vi "ZVisualize_SingleArrayTesting.vi"() -> ()   [LabVIEW 2016]
uses:
  subVI/ZDataVIS_StateWire.ctl
  <vilib>/Utility/miscctls.llb/LVPointDoubleTypeDef.ctl
panel:
  in  "X Scale Selection":enum32{"Manual", "Auto"}(tab)=enum."Auto"
  in  "Manual CTLs":T1={"X Low"=-0.2, "X High"=-0.1, "X Step Size"=0.001} {"X Step Size" format="%#_6p"; "X High" format="%#_6p"; "X Low" format="%#_6p"}
  in  "Auto CTLs":cluster{"METHOD":bool, "Steps":dbl}={"METHOD"=FALSE, "Steps"=100.0}
  out "XY Graph":cluster{dbl[], dbl[]}[](graph)
  out "Field":dbl=4.108108108108109
  out "slowest":dbl=7.00003046875
  out "2term Intensity":dbl[][](graph)
  in  "X Axis":T2(ring)=enum."dI/dV 2T"
  in  "Y Axis":T2(ring)
  in  "Fake Point Value":dbl format="%#_13g"
  in  "Filter retrieved data? 2":bool=TRUE
  in  "stop":bool
  in  "side points 4T 2":i32=8
  out "side points 4Ttemp":i32=8
  in  "side points 2T 2":i32=12
  out "side points 2Ttemp":i32=12
  in  "side points 4T":i32=8
  in  "side points 2T":i32=12
  in  "Fit Points 2":dbl=10.0
  in  "T/B     third axis":bool
  in  "color scale":u32[](array[colorbox])=[16711680, 16772608, 6618880, 3381759, 16860, 10420479]
  in  "Voffset -2T":dbl=2e-05 format="%#_6p"
  in  "Voffset-4T":dbl=-5e-05 format="%#_4p"
  in  "Field/Temperature":i32(slide) min=0 max=36 step=1
  out "Scan names":string[](array[string])=["DAQ_Vbg", "B", "B"]
  out "Cursor Graph":cluster{dbl[], dbl[]}(graph)={[0.0, 0.0, 0.0, 0.0, 0.0, 0.0, 0.0, 0.0, 0.25, 0.25, 0.25, 0.25, 0.25, 0.25, 0.25, 0.25, 0.5, 0.5, 0.5, 0.5, 0.5, 0.5, 0.5, 0.5, 0.75, 0.75, 0.75, 0.75, 0.75, 0.75, 0.75, 0.75, 1.0, 1.0, 1.0, 1.0, 1.0, 1.0, 1.0, 1.0, 1.25, 1.25, 1.25, 1.25, 1.25, 1.25, 1.25, 1.25, 1.5, 1.5, 1.5, 1.5, 1.5, 1.5, 1.5, 1.5, 1.75, 1.75, 1.75, 1.75, 1.75, 1.75, 1.75, 1.75, 2.0, 2.0, 2.0, 2.0, 2.0, 2.0, 2.0, 2.0, 2.25, 2.25, 2.25, 2.25, 2.25, 2.25, 2.25, 2.25, 2.5, 2.5, 2.5, 2.5, 2.5, 2.5, 2.5, 2.5, 2.75, 2.75, 2.75, 2.75, 2.75, 2.75, 2.75, 2.75, 3.0, 3.0, 3.0, 3.0, 3.0, 3.0, 3.0, 3.0, 3.25, 3.25, 3.25, 3.25, 3.25, 3.25, 3.25, 3.25, 3.5, 3.5, 3.5, 3.5, 3.5, 3.5, 3.5, 3.5, 3.75, 3.75, 3.75, 3.75, 3.75, 3.75, 3.75, 3.75, 4.0, 4.0, 4.0, 4.0, 4.0, 4.0, 4.0, 4.0, 4.25, 4.25, 4.25, 4.25, 4.25, 4.25, 4.25, 4.25, 4.5, 4.5, 4.5, 4.5, 4.5, 4.5, 4.5, 4.5, 4.75, 4.75, 4.75, 4.75, 4.75, 4.75, 4.75, 4.75, 5.0, 5.0, 5.0, 5.0, 5.0, 5.0, 5.0, 5.0, 5.25, 5.25, 5.25, 5.25, 5.25, 5.25, 5.25, 5.25, 5.5, 5.5, 5.5, 5.5, 5.5, 5.5, 5.5, 5.5, 5.75, 5.75, 5.75, 5.75, 5.75, 5.75, 5.75, 5.75, 6.0, 6.0, 6.0, 6.0, 6.0, 6.0, 6.0, 6.0, 6.25, 6.25, 6.25, 6.25, 6.25, 6.25, 6.25, 6.25, 6.5, 6.5, 6.5, 6.5, 6.5, 6.5, 6.5, 6.5, 6.75, 6.75, 6.75, 6.75, 6.75, 6.75, 6.75, 6.75, 7.0, 7.0, 7.0, 7.0, 7.0, 7.0, 7.0, 7.0, 7.25, 7.25, 7.25, 7.25, 7.25, 7.25, 7.25, 7.25, 7.5, 7.5, 7.5, 7.5, 7.5, 7.5, 7.5, 7.5, 7.75, 7.75, 7.75, 7.75, 7.75, 7.75, 7.75, 7.75, 8.0, 8.0, 8.0, 8.0, 8.0, 8.0, 8.0, 8.0, 8.25, 8.25, 8.25, 8.25, 8.25, 8.25, 8.25, 8.25, 8.5, 8.5, 8.5, 8.5, 8.5, 8.5, 8.5, 8.5, 8.75, 8.75, 8.75, 8.75, 8.75, 8.75, 8.75, 8.75, 9.0, 9.0, 9.0, 9.0, 9.0, 9.0, 9.0, 9.0, 9.25, 9.25, 9.25, 9.25, 9.25, 9.25, 9.25, 9.25, 9.5, 9.5, 9.5, 9.5, 9.5, 9.5, 9.5, 9.5, 9.75, 9.75, 9.75, 9.75, 9.75, 9.75, 9.75, 9.75, 10.0, 10.0, 10.0, 10.0, 10.0, 10.0, 10.0, 10.0, 10.25, 10.25, 10.25, 10.25, 10.25, 10.25, 10.25, 10.25, 10.5, 10.5, 10.5, 10.5, 10.5, 10.5, 10.5, 10.5, 10.75, 10.75, 10.75, 10.75, 10.75, 10.75, 10.75, 10.75, 11.0, 11.0, 11.0, 11.0, 11.0, 11.0, 11.0, 11.0, 11.25, 11.25, 11.25, 11.25, 11.25, 11.25, 11.25, 11.25, 11.5, 11.5, 11.5, 11.5, 11.5, 11.5, 11.5, 11.5, 11.75, 11.75, 11.75, 11.75, 11.75, 11.75, 11.75, 11.75, 12.0, 12.0, 12.0, 12.0, 12.0, 12.0, 12.0, 12.0, 12.25, 12.25, 12.25, 12.25, 12.25, 12.25, 12.25, 12.25, 12.5, 12.5, 12.5, 12.5, 12.5, 12.5, 12.5, 12.5, 12.75, 12.75, 12.75, 12.75, 12.75, 12.75, 12.75, 12.75, 13.0, 13.0, 13.0, 13.0, 13.0, 13.0, 13.0, 13.0, 13.25, 13.25, 13.25, 13.25, 13.25, 13.25, 13.25, 13.25, 13.5, 13.5, 13.5, 13.5, 13.5, 13.5, 13.5, 13.5, 13.75, 13.75, 13.75, 13.75, 13.75, 13.75, 13.75, 13.75, 14.0, 14.0, 14.0, 14.0, 14.0, 14.0, 14.0, 14.0, 14.25, 14.25, 14.25, 14.25, 14.25, 14.25, 14.25, 14.25, 14.5, 14.5, 14.5, 14.5, 14.5, 14.5, 14.5, 14.5, 14.75, 14.75, 14.75, 14.75, 14.75, 14.75, 14.75, 14.75, 15.0, 15.0, 15.0, 15.0, 15.0, 15.0, 15.0, 15.0], [0.0, 1.0, 2.0, 3.0, 4.0, 5.0, 6.0, 7.0, 0.0, 1.0, 2.0, 3.0, 4.0, 5.0, 6.0, 7.0, 0.0, 1.0, 2.0, 3.0, 4.0, 5.0, 6.0, 7.0, 0.0, 1.0, 2.0, 3.0, 4.0, 5.0, 6.0, 7.0, 0.0, 1.0, 2.0, 3.0, 4.0, 5.0, 6.0, 7.0, 0.0, 1.0, 2.0, 3.0, 4.0, 5.0, 6.0, 7.0, 0.0, 1.0, 2.0, 3.0, 4.0, 5.0, 6.0, 7.0, 0.0, 1.0, 2.0, 3.0, 4.0, 5.0, 6.0, 7.0, 0.0, 1.0, 2.0, 3.0, 4.0, 5.0, 6.0, 7.0, 0.0, 1.0, 2.0, 3.0, 4.0, 5.0, 6.0, 7.0, 0.0, 1.0, 2.0, 3.0, 4.0, 5.0, 6.0, 7.0, 0.0, 1.0, 2.0, 3.0, 4.0, 5.0, 6.0, 7.0, 0.0, 1.0, 2.0, 3.0, 4.0, 5.0, 6.0, 7.0, 0.0, 1.0, 2.0, 3.0, 4.0, 5.0, 6.0, 7.0, 0.0, 1.0, 2.0, 3.0, 4.0, 5.0, 6.0, 7.0, 0.0, 1.0, 2.0, 3.0, 4.0, 5.0, 6.0, 7.0, 0.0, 1.0, 2.0, 3.0, 4.0, 5.0, 6.0, 7.0, 0.0, 1.0, 2.0, 3.0, 4.0, 5.0, 6.0, 7.0, 0.0, 1.0, 2.0, 3.0, 4.0, 5.0, 6.0, 7.0, 0.0, 1.0, 2.0, 3.0, 4.0, 5.0, 6.0, 7.0, 0.0, 1.0, 2.0, 3.0, 4.0, 5.0, 6.0, 7.0, 0.0, 1.0, 2.0, 3.0, 4.0, 5.0, 6.0, 7.0, 0.0, 1.0, 2.0, 3.0, 4.0, 5.0, 6.0, 7.0, 0.0, 1.0, 2.0, 3.0, 4.0, 5.0, 6.0, 7.0, 0.0, 1.0, 2.0, 3.0, 4.0, 5.0, 6.0, 7.0, 0.0, 1.0, 2.0, 3.0, 4.0, 5.0, 6.0, 7.0, 0.0, 1.0, 2.0, 3.0, 4.0, 5.0, 6.0, 7.0, 0.0, 1.0, 2.0, 3.0, 4.0, 5.0, 6.0, 7.0, 0.0, 1.0, 2.0, 3.0, 4.0, 5.0, 6.0, 7.0, 0.0, 1.0, 2.0, 3.0, 4.0, 5.0, 6.0, 7.0, 0.0, 1.0, 2.0, 3.0, 4.0, 5.0, 6.0, 7.0, 0.0, 1.0, 2.0, 3.0, 4.0, 5.0, 6.0, 7.0, 0.0, 1.0, 2.0, 3.0, 4.0, 5.0, 6.0, 7.0, 0.0, 1.0, 2.0, 3.0, 4.0, 5.0, 6.0, 7.0, 0.0, 1.0, 2.0, 3.0, 4.0, 5.0, 6.0, 7.0, 0.0, 1.0, 2.0, 3.0, 4.0, 5.0, 6.0, 7.0, 0.0, 1.0, 2.0, 3.0, 4.0, 5.0, 6.0, 7.0, 0.0, 1.0, 2.0, 3.0, 4.0, 5.0, 6.0, 7.0, 0.0, 1.0, 2.0, 3.0, 4.0, 5.0, 6.0, 7.0, 0.0, 1.0, 2.0, 3.0, 4.0, 5.0, 6.0, 7.0, 0.0, 1.0, 2.0, 3.0, 4.0, 5.0, 6.0, 7.0, 0.0, 1.0, 2.0, 3.0, 4.0, 5.0, 6.0, 7.0, 0.0, 1.0, 2.0, 3.0, 4.0, 5.0, 6.0, 7.0, 0.0, 1.0, 2.0, 3.0, 4.0, 5.0, 6.0, 7.0, 0.0, 1.0, 2.0, 3.0, 4.0, 5.0, 6.0, 7.0, 0.0, 1.0, 2.0, 3.0, 4.0, 5.0, 6.0, 7.0, 0.0, 1.0, 2.0, 3.0, 4.0, 5.0, 6.0, 7.0, 0.0, 1.0, 2.0, 3.0, 4.0, 5.0, 6.0, 7.0, 0.0, 1.0, 2.0, 3.0, 4.0, 5.0, 6.0, 7.0, 0.0, 1.0, 2.0, 3.0, 4.0, 5.0, 6.0, 7.0, 0.0, 1.0, 2.0, 3.0, 4.0, 5.0, 6.0, 7.0, 0.0, 1.0, 2.0, 3.0, 4.0, 5.0, 6.0, 7.0, 0.0, 1.0, 2.0, 3.0, 4.0, 5.0, 6.0, 7.0, 0.0, 1.0, 2.0, 3.0, 4.0, 5.0, 6.0, 7.0, 0.0, 1.0, 2.0, 3.0, 4.0, 5.0, 6.0, 7.0, 0.0, 1.0, 2.0, 3.0, 4.0, 5.0, 6.0, 7.0, 0.0, 1.0, 2.0, 3.0, 4.0, 5.0, 6.0, 7.0, 0.0, 1.0, 2.0, 3.0, 4.0, 5.0, 6.0, 7.0, 0.0, 1.0, 2.0, 3.0, 4.0, 5.0, 6.0, 7.0, 0.0, 1.0, 2.0, 3.0, 4.0, 5.0, 6.0, 7.0, 0.0, 1.0, 2.0, 3.0, 4.0, 5.0, 6.0, 7.0]}
  in  "Fit Points":dbl=10.0
  in  "file path (use dialog)":path=path "B:/SketchSET/SA03008H.20180718/processed/51-B+BG_0to15_0.25steps_@0-7T_1step_at.2Hz.dat"
  in  "OK":bool
  # "VS"
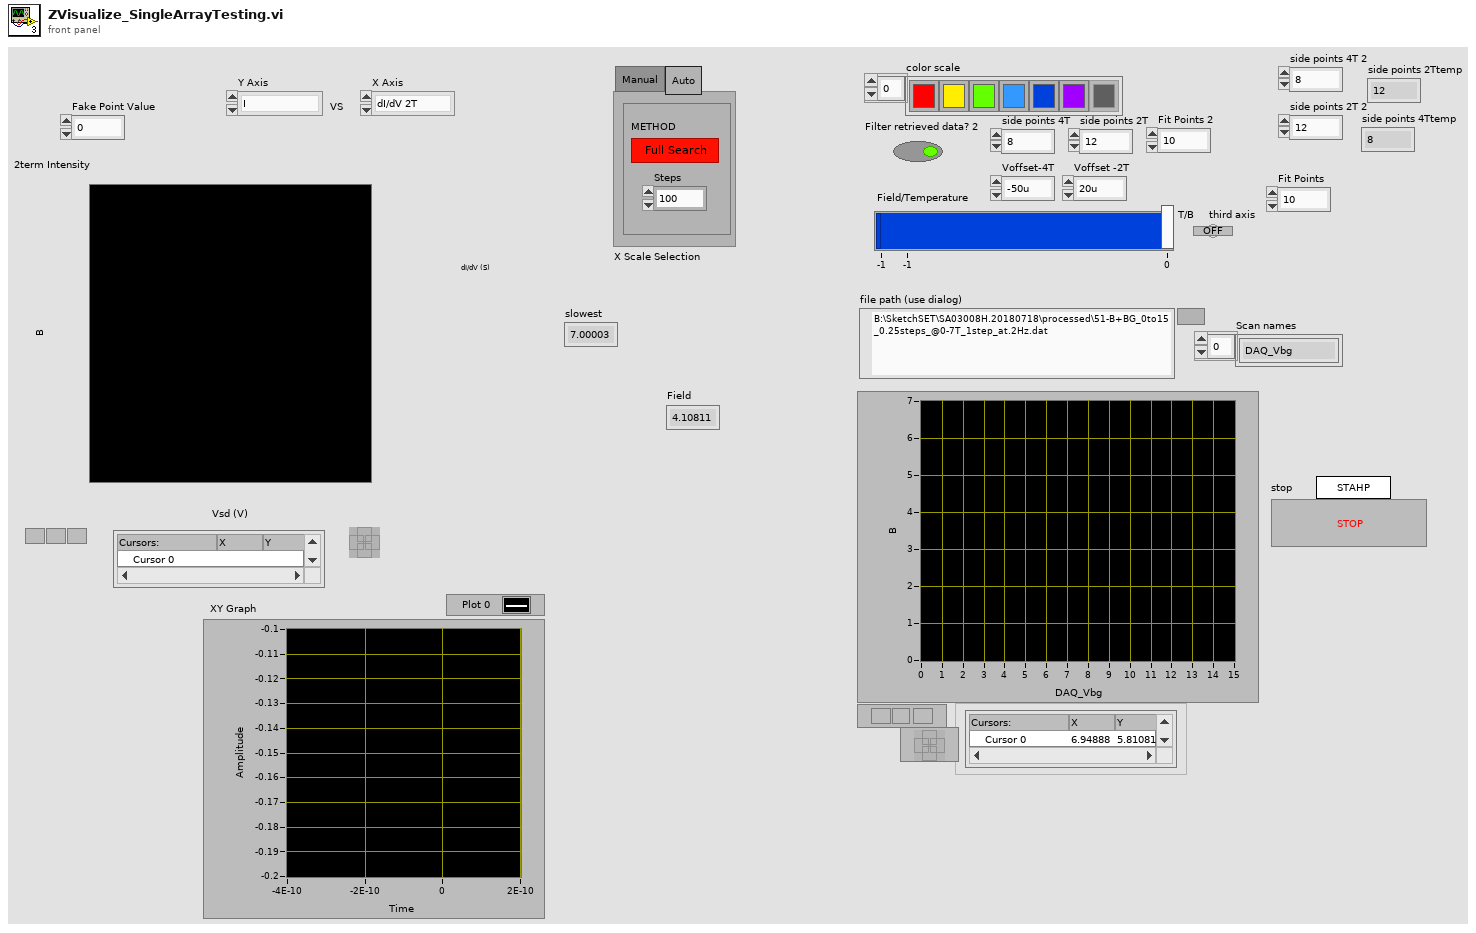
[diagram p1: front panel]
types:
  T1 = cluster{"X Low":dbl, "X High":dbl, "X Step Size":dbl}
  T2 = enum16{"I", "Vsd", "V4T", "dI/dV 2T", "dV/dI 2T", "dV/dI 4T", "dI/dV 4T"}
  T3 = enum32{"invalid app kind", "Development System", "Run Time System", "Student Edition", "Embedded LabVIEW", "Evaluation", "Custom"}
  T4 = cluster{"I":dbl[], "Vsd":dbl[], "V4T":dbl[], "dI/dV 2T":dbl[], "dV/dI 2T":dbl[], "dV/dI 4T":dbl[], "dI/dV 4T":dbl[]}[][][]
  T5 = enum32{"Invalid", "Standard", "Closed", "Hidden", "Minimized", "Maximized"}
  T6 = typedef "ZDataVIS_StateWire.ctl" = cluster{"Core":cluster{"Current VI Reference":refnum<vi>, "Close Panel on Exit?":bool}, "Sweep Data Cluster":cluster{"Vfast":dbl[][], "Vslow":dbl[], "Vslowest":dbl[], "Comments":string, "Scan names":string[]}, "Cursor Info":cluster{"Fast Index":dbl[], "Slow Index":dbl, "Slow Indices":dbl[], "Raw Cursor Position":T7, "Field / temp":i32}, "Scan names":string[], "Data DVR":refnum<data-value>}
  T7 = typedef "LVPointDoubleTypeDef.ctl" = cluster{"X":dbl, "Y":dbl}
  T8 = cluster{"Fast Index (Cursor X)":dbl[], "Slow Index (Cursor Y)":dbl, "Slow Indices":dbl[], "Raw Cursor Position":T7}
  T9 = cluster{"Vfast":dbl[][], "Vslow":dbl[], "Vslowest":dbl[], "Comments":string, "Scan names":string[]}
  T10 = cluster{"Current VI Reference":refnum<vi>, "Close Panel on Exit?":bool}
  T11 = cluster{"IV":cluster{dbl[], dbl[]}[][][], "IV-2T":cluster{dbl[], dbl[]}[][][], "Vfast":dbl[][], "Vslow":dbl[], "Vslowest":dbl[], "Comments":string, "Scan names":string[]}[]
  T12 = cluster{"IV":cluster{dbl[], dbl[]}[][][], "IV-2T":cluster{dbl[], dbl[]}[][][], "Vfast":dbl[][], "Vslow":dbl[], "Vslowest":dbl[], "Comments":string, "Scan names":string[]}
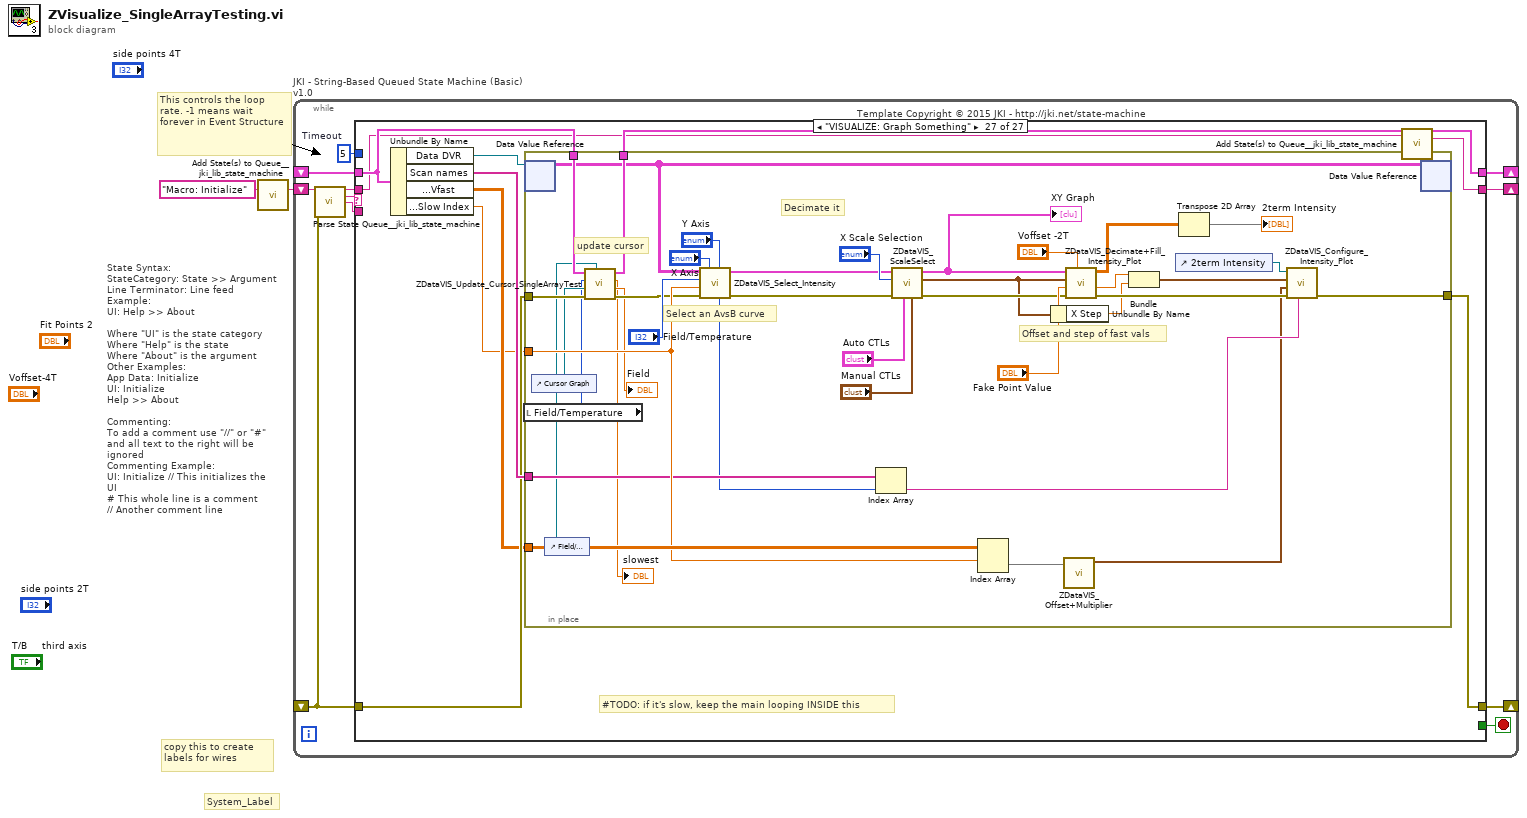
[diagram p0: block diagram]
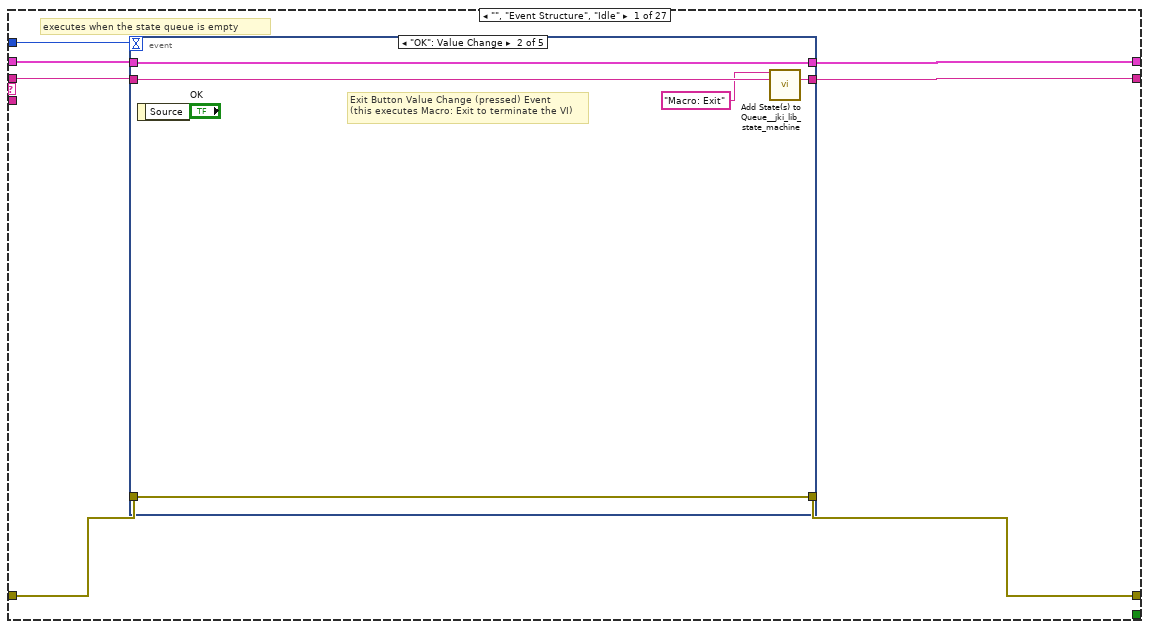
[diagram p2: hidden frame]
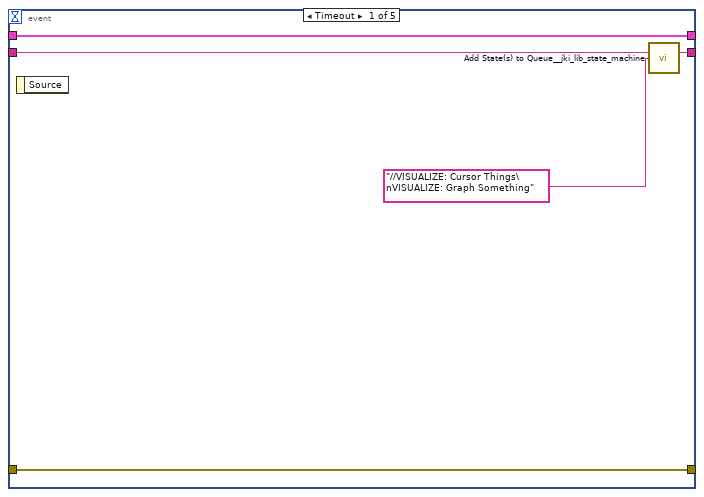
[diagram p3: hidden frame]
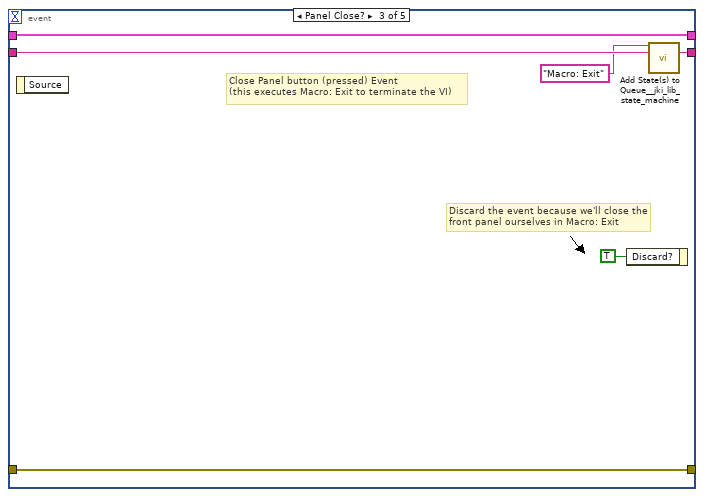
[diagram p4: hidden frame]
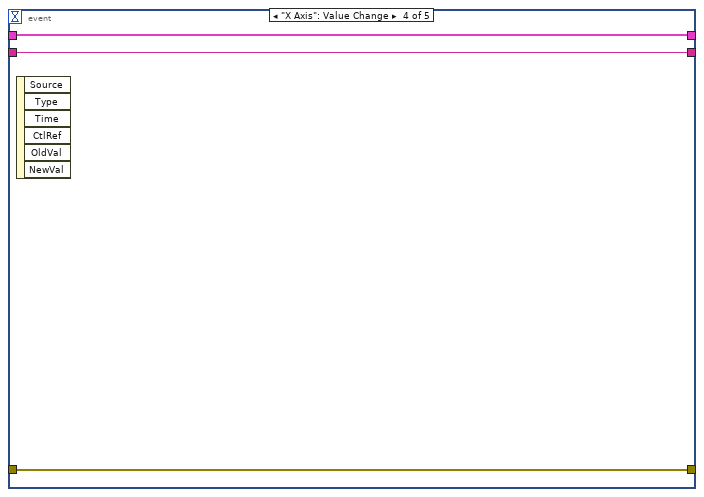
[diagram p5: hidden frame]
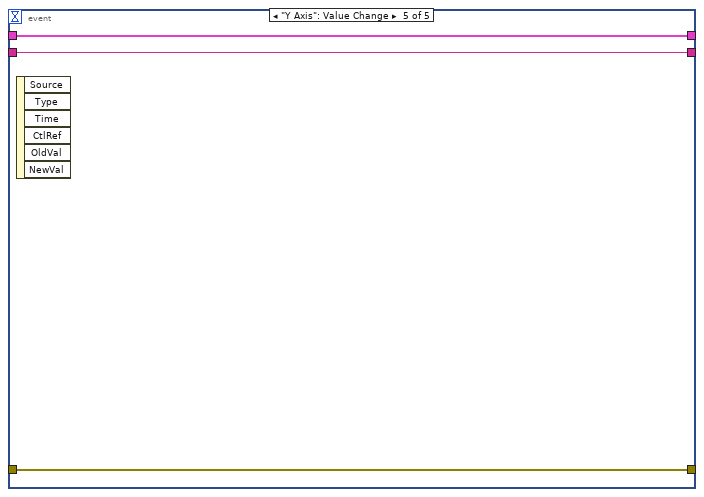
[diagram p6: hidden frame]
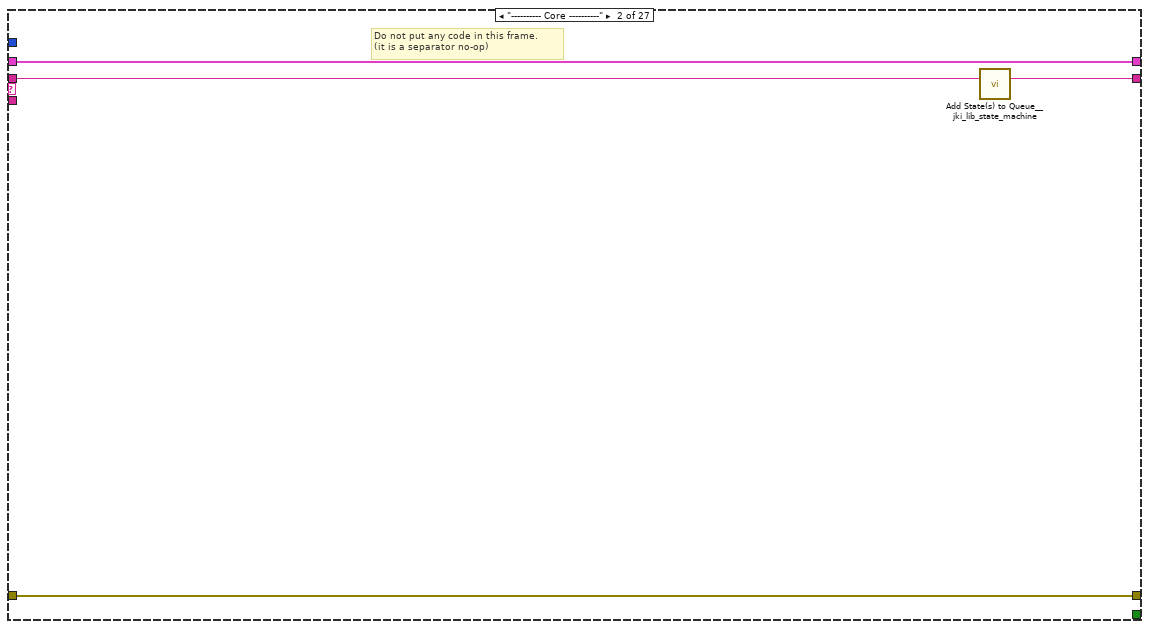
[diagram p7: hidden frame]
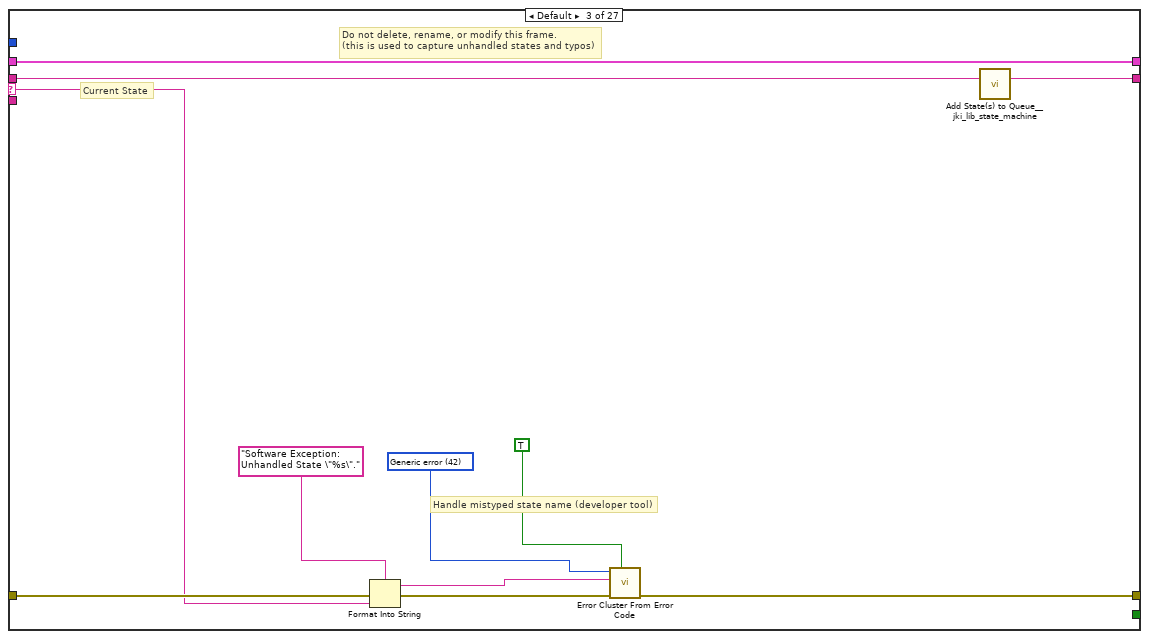
[diagram p8: hidden frame]
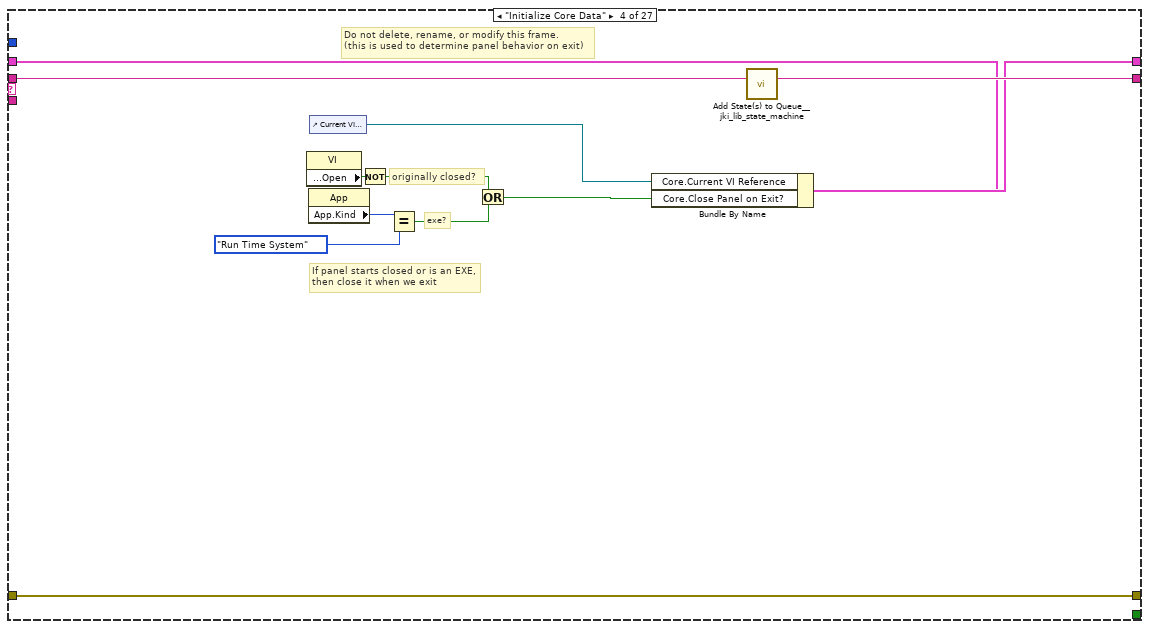
[diagram p9: hidden frame]
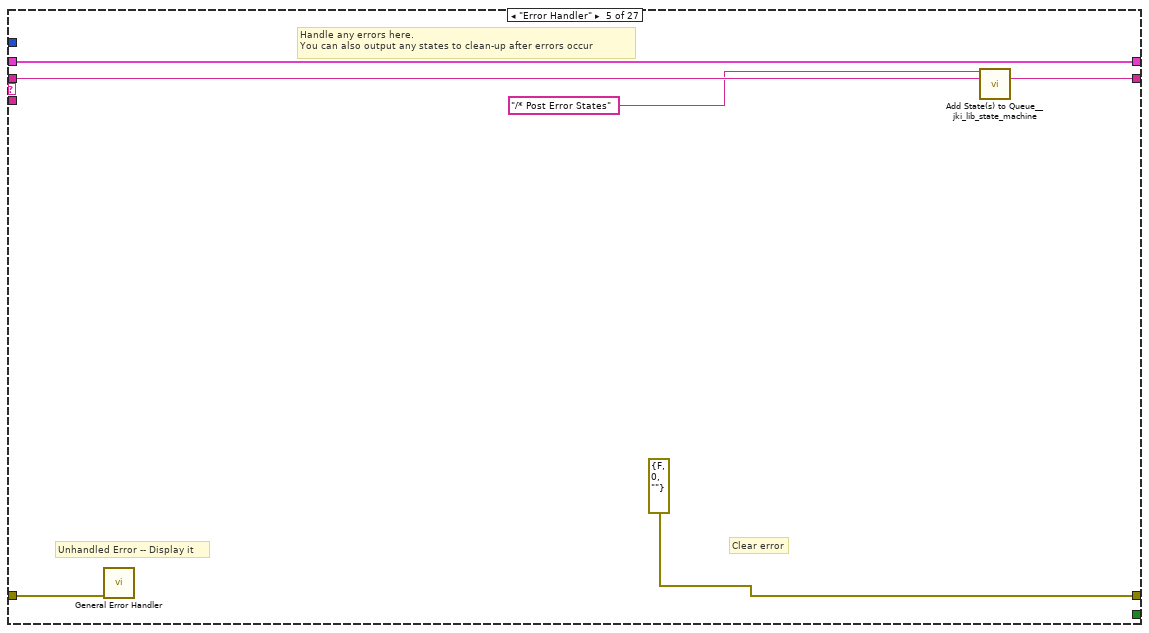
[diagram p10: hidden frame]
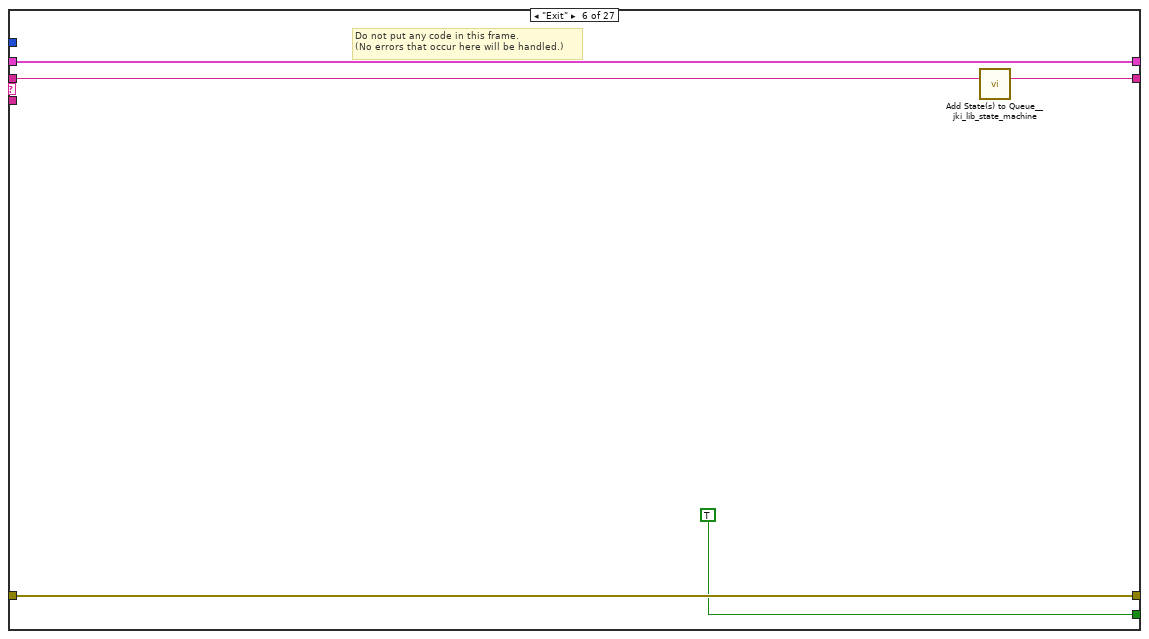
[diagram p11: hidden frame]
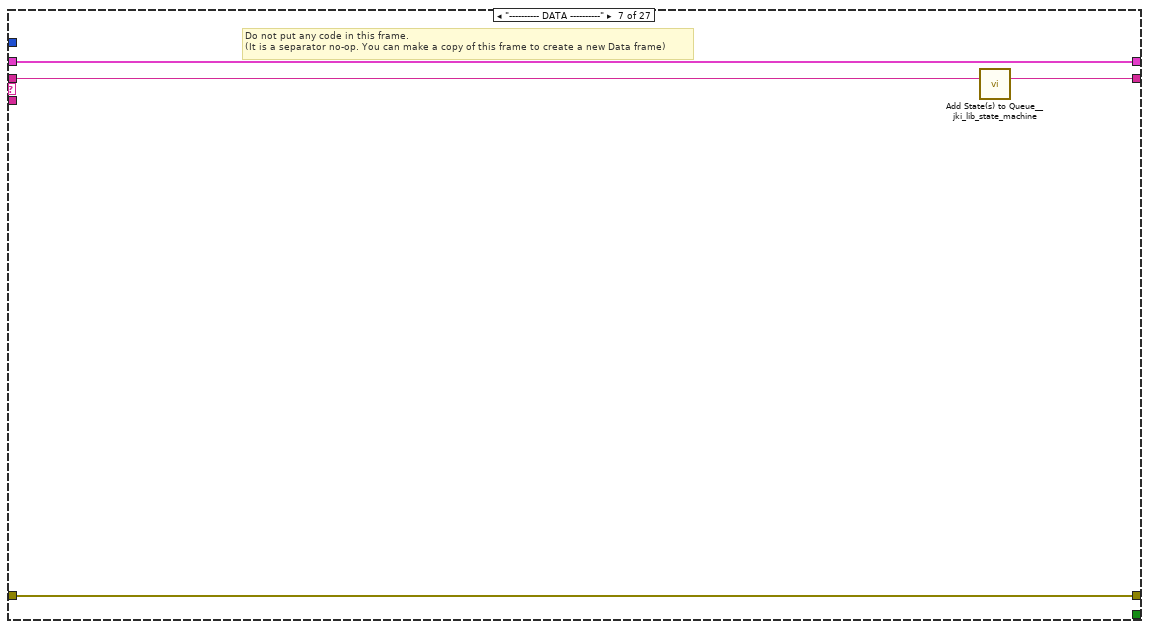
[diagram p12: hidden frame]
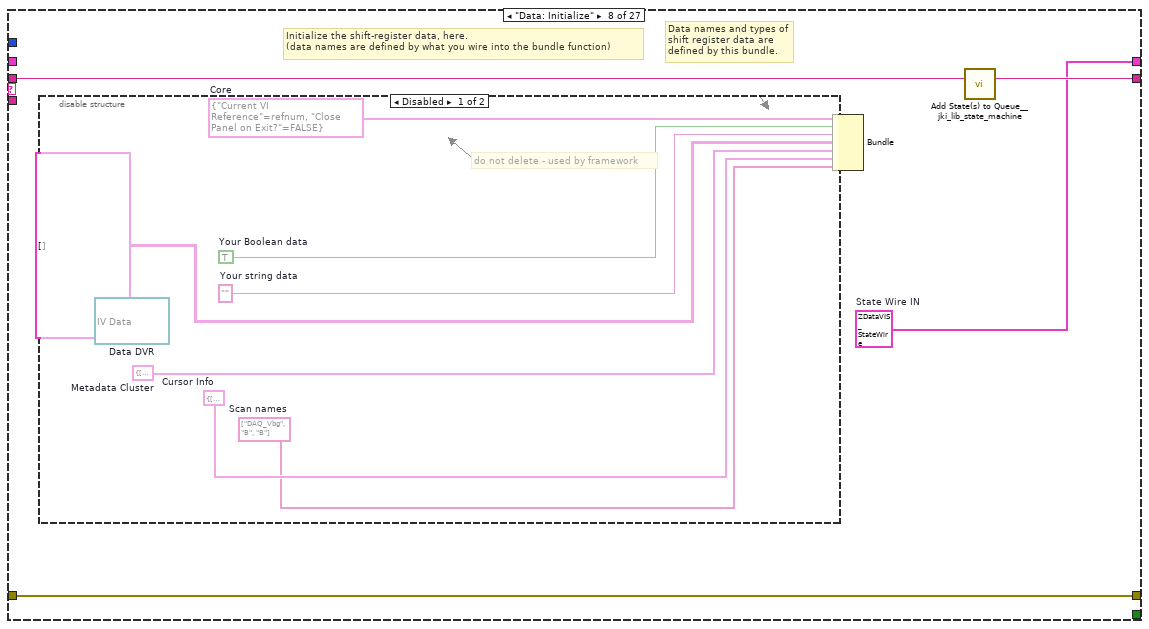
[diagram p13: hidden frame]
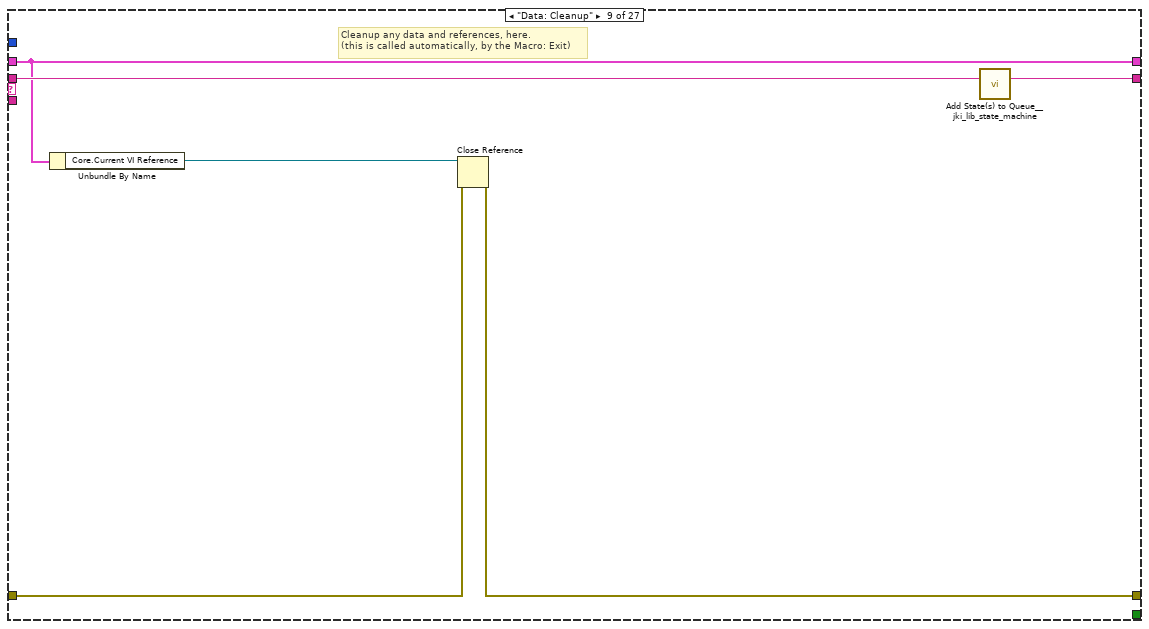
[diagram p15: hidden frame]
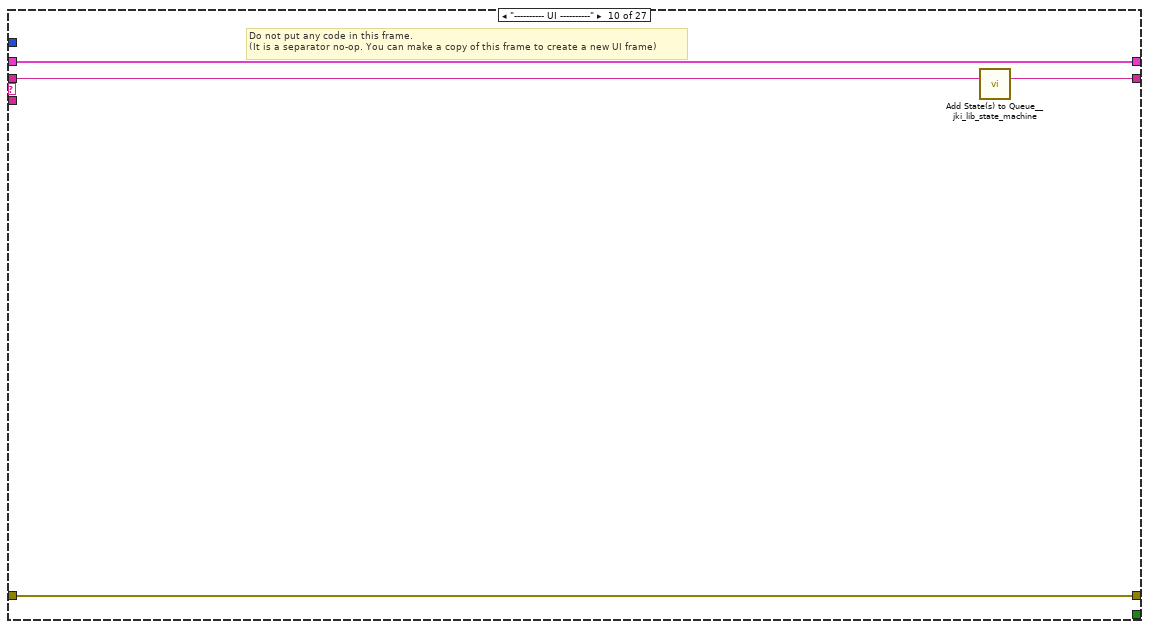
[diagram p16: hidden frame]
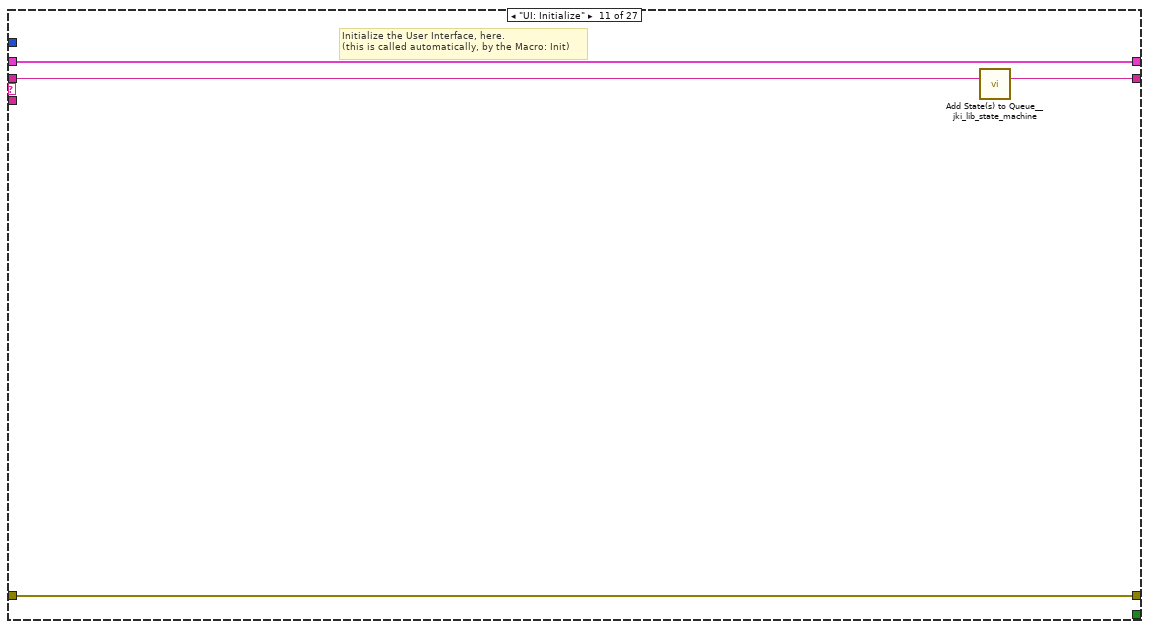
[diagram p17: hidden frame]
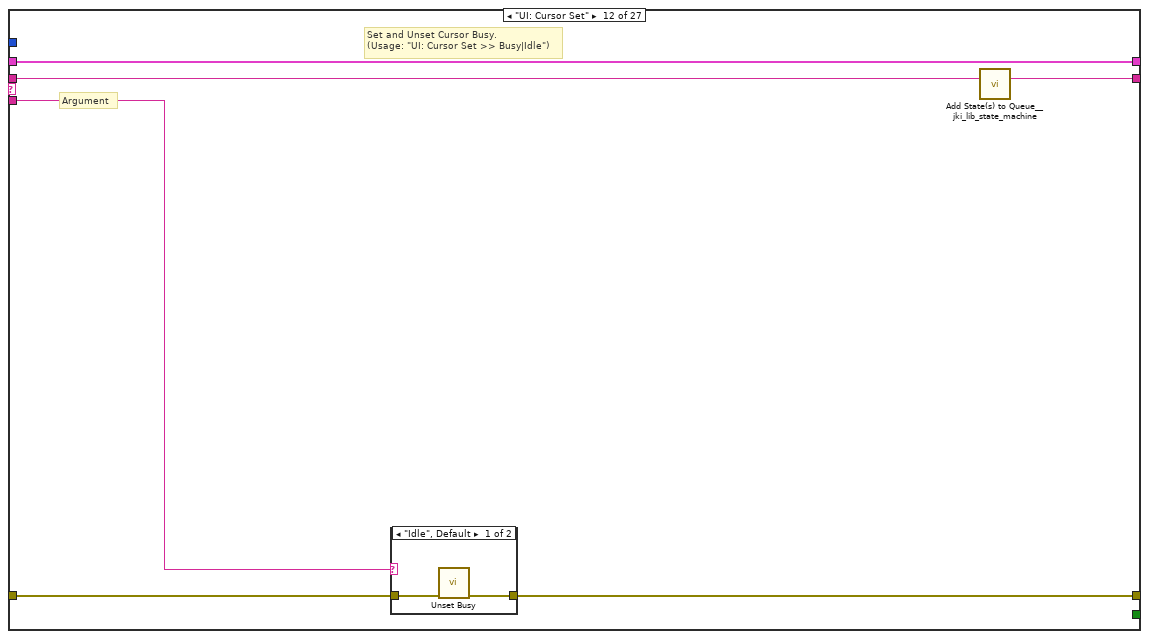
[diagram p18: hidden frame]
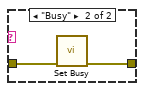
[diagram p19: hidden frame]
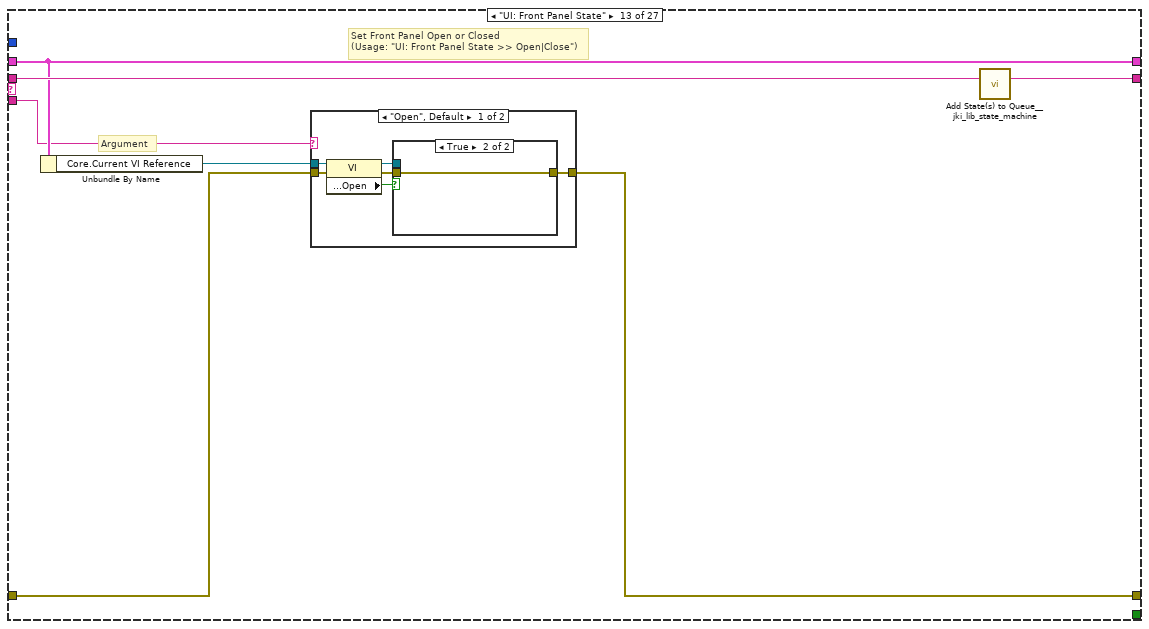
[diagram p20: hidden frame]
diagram:
  # "State Syntax:\nStateCategory: State >> Argument\nLine Terminator: Line feed\nExample:\nUI: Help >> About\n\nWhere \"UI\" is the state category\nWhere \"Help\" is the state\nWhere \"About\" is the argument\nOther Examples:\nApp Data: Initialize\nUI: Initialize\nHelp >> About\n\nCommenting:\nTo add a comment use \"//\" or \"#\" and all text to the right will be ignored\nCommenting Example:\nUI: Initialize // This initializes the UI\n# This whole line is a comment\n// Another comment line"
  # "copy this to create labels for wires"
  # "This controls the loop rate. -1 means wait forever in Event Structure"
  # "System_Label"
  n1 = call <vilib>:"Add State(s) to Queue__jki_lib_state_machine.vi"("State(s) in (\"\")"="Macro: Initialize") -> ("States Out"=w2:string)  [unwired: 14 in]
  n2 = while "JKI - String-Based Queued State Machine (Basic) v1.0" {
    shift-right: [w6] -> _
    shift-left: _ -> [w5]
    shift-right: [w9] -> _
    shift-left: _ -> [w3]
    shift-right: [w8] -> _
    shift-left: w2 -> [w10]
    stop <- w7 stop-if-true
    w4 = 5  # Timeout
    # "Template Copyright © 2015 JKI - http://jki.net/state-machine"
    n3 = call <vilib>:"Parse State Queue__jki_lib_state_machine.vi"("State Queue"=w10, "Error In (no error)"=w3) -> ("Remaining States"=w12:string, "Current State"=w13:string, "Arguments"=w11:string)  [unwired: 11 in]
    n4 = case shown="\"VISUALIZE: Graph Something\"" w13 {
      selector: w13 -> [_ _ w47 _ _ _ _ _ _ _ _ _ _ _ _ _ _ _ _ _ _ _ _ _ _ _ _]
      tunnel: w12 -> [w20 w46 w51 w69 w75 w80 w84 w88 w101 w105 w109 w115 w126 w152 w157 w167 w172 w183 w187 w209 w213 w217 w235 w249 w253 w265 w296]
      tunnel: w11 -> [_ _ _ _ _ _ _ _ _ _ _ w110 w120 _ _ _ _ _ _ _ _ _ _ _ _ _ _]
      tunnel: w5 -> [w18 w43 w49 w60 w72 w78 w81 _ w96 w102 w107 w113 w122 w149 w154 w164 w169 w180 w184 w203 w210 w214 w233 w246 w250 w255 w297]
      tunnel: [w17 w44 w53 w66 errorcluster {"status"=FALSE, "code"=0, "source"=""} ("error out") w77 w82 w86 w97 w103 w106 w111 w123 w150 w155 w165 w170 w181 w185 w201 w211 w215 w218 w247 w251 w263 w299] -> w9
      tunnel: w3 -> [w16 w44 w52 w66 w71 w77 w82 w86 w98 w103 w106 w112 w124 w150 w155 w165 w170 w181 w185 w206 w211 w215 w219 w247 w251 w263 w300]
      tunnel: [w19 w45 w50 w68 w74 w79 w83 w87 w100 w104 w108 w114 w125 w151 w156 w166 w171 w182 w186 w208 w212 w216 w234 w248 w252 w264 w295] -> w8
      tunnel: [_ _ _ _ _ TRUE _ _ _ _ _ _ _ _ _ _ _ _ _ _ _ _ _ _ _ _ _] -> w7
      tunnel: [w15 w43 w49 w67 w72 w78 w81 w85 w96 w102 w107 w113 w122 w149 w154 w164 w169 w180 w184 w202 w210 w214 w233 w246 w250 w254 w298] -> w6
      tunnel: w4 -> [w14 _ _ _ _ _ _ _ _ _ _ _ _ _ _ _ _ _ _ _ _ _ _ _ _ _ _]
      frame "", "Event Structure", "Idle" {
        # "executes when the state queue is empty"
        n5 = event shown="[1] \"OK\": Value Change" {
          selector: _ -> [_ _ _ _ _]
          dyn-events: _ -> [_ _ _ _ _]
          timeout: w14 -> [_ _ _ _ _]
          tunnel: w20 -> [w25 w30 w36 w38 w41]
          tunnel: [w24 w29 w35 w38 w41] -> w19
          tunnel: w18 -> [w22 w27 w33 w39 w42]
          tunnel: [w23 w28 w34 w37 w40] -> w17
          tunnel: w16 -> [w23 w28 w34 w37 w40]
          tunnel: [w22 w27 w33 w39 w42] -> w15
          event Timeout {
            n6 = event-data() -> ()  [unwired: 1 in, 1 out]
            n7 = call <vilib>:"Add State(s) to Queue__jki_lib_state_machine.vi"("State(s) in (\"\")"=w25, "State(s) at Back (\"\")"="//VISUALIZE: Cursor Things\nVISUALIZE: Graph Something" ("State(s) at Back (\"\")")) -> ("States Out"=w24:string)  [unwired: 13 in]
          }
          event "OK": Value Change {
            # "Exit Button Value Change (pressed) Event\n(this executes Macro: Exit to terminate the VI)"
            n8 = event-data() -> ()  [unwired: 1 in, 1 out]
            n9 = call <vilib>:"Add State(s) to Queue__jki_lib_state_machine.vi"("State(s) in Front (\"\")"="Macro: Exit", "State(s) in (\"\")"=w30) -> ("States Out"=w29:string)  [unwired: 13 in]
          }
          event Panel Close? {
            # "Discard the event because we'll close the front panel ourselves in Macro: Exit"
            # "Close Panel button (pressed) Event\n(this executes Macro: Exit to terminate the VI)"
            n10 = event-data() -> ()  [unwired: 1 in, 1 out]
            n11 = event-data("Discard?"=TRUE) -> ()  [unwired: 1 in, 1 out]
            n12 = call <vilib>:"Add State(s) to Queue__jki_lib_state_machine.vi"("State(s) in Front (\"\")"="Macro: Exit", "State(s) in (\"\")"=w36) -> ("States Out"=w35:string)  [unwired: 13 in]
          }
          event "X Axis": Value Change {
            n13 = event-data() -> ()  [unwired: 1 in, 6 out]
          }
          event "Y Axis": Value Change {
            n14 = event-data() -> ()  [unwired: 1 in, 6 out]
          }
        }
      }
      frame "---------- Core ----------" {
        # "Do not put any code in this frame.\n(it is a separator no-op)"
        n15 = call <vilib>:"Add State(s) to Queue__jki_lib_state_machine.vi"("State(s) in (\"\")"=w46) -> ("States Out"=w45:string)  [unwired: 14 in]
      }
      frame Default {
        w56 = 42 items=["No error", "Argument error", "Memory is full", "Out of zone", "End of file", "File already open", "Generic file I/O error", "File not found", "File permission error", "Disk is full", "Duplicate path", "Too many files open", "System feature not enabled", "Resource file not found", "Cannot add resource", "Resource not found", "Image not found", "Image memory error", "Pen does not exist", "Config type invalid", "Config token not found", "Config parse error", "Config memory error", "Bad external code format", "Bad external code offset", "External code not present", "Null window", "Destroy window error", "Null menu", "Print aborted", "Bad print record", "Print driver error", "Windows error during printing", "Memory error during printing", "Print dialog error", "Generic print error", "Invalid device refnum", "Device not found", "Device parameter error", "Device unit error", "Cannot open device", "Device call aborted", "Generic error", "Cancelled by user", "Object ID too low", "Object ID too high", "Object not in heap", "Unknown heap", "Unknown object (invalid DefProc)", "Unknown object (DefProc not in table)", "Message out of range", "Invalid (null) method", "Unknown message", "Manager call not supported", "Bad address", "Network operation in progress", "Network operation timed out", "Connection is busy", "Network attribute not supported", "Network error", "Address in use", "System out of memory", "Connection aborted", "Connection refused", "Not connected", "Already connected", "Connection closed", "Initialization error (interapplication manager)", "Bad occurrence", "Wait on unbound occurrence handler", "Occurrence queue overflow", "Datalog type conflict", "Unused", "Unrecognized type (interapplication manager)", "Memory corrupt", "Failed to make temporary DLL", "Old CIN version", "Drag socket not found", "Failed to load drop-object", "Failed to register OLE object", "Failed to release OLE object", "Format specifier type mismatch", "Unknown format specifier", "Too few format specifiers", "Too many format specifiers", "Scan failed", "Newer CIN version", "Error converting to variant", "Runtime menu error", "Password tampered", "Variant attribute not found", "Incompatible variant data type", "Event data is not available", "Event Store is not present", "Occurrence is not found", "Event Queue is not created", "Event info is not available", "Refnum passed is NULL", "Error retrieving Class GUID", "Error retrieving CoClass GUID", "Error retrieving TypeLib GUID.", "Bad built application magic bytes.", "Specific driver is different from the specific driver associated with the Logical Name.", "There is no session opened to the class driver.", "Max Error", "MAX - Error with config objects", "MAX - Error loading configuration", "MAX - Group not supported"]
        # "Current State"
        # "Do not delete, rename, or modify this frame.\n(this is used to capture unhandled states and typos)"
        # "Handle mistyped state name (developer tool)"
        n16 = Format Into String(format string="Software Exception: Unhandled State \"%s\"." ("message"), error in=w52, w47) -> (resulting string=w55:string, error out=w54:errorcluster)  [unwired: 1 in]
        n17 = call <vilib>:"Error Cluster From Error Code.vi"("show call chain? (False)"=TRUE, "error in (no error)"=w54, "error message (\"\")"=w55, "error code (0)"=w56) -> ("error out"=w53:errorcluster)  [unwired: 5 in]
        n18 = call <vilib>:"Add State(s) to Queue__jki_lib_state_machine.vi"("State(s) in (\"\")"=w51) -> ("States Out"=w50:string)  [unwired: 14 in]
      }
      frame "Initialize Core Data" {
        # "Do not delete, rename, or modify this frame.\n(this is used to determine panel behavior on exit)"
        # "originally closed?"
        # "exe?"
        # "If panel starts closed or is an EXE, then close it when we exit"
        n19 = property class="VI"() -> ("Front Panel.Open"=w65:bool)  [unwired: 2 in, 2 out]
        n20 = property class="App"() -> ("App.Kind"=w64:T3)  [unwired: 2 in, 2 out]
        n21 = control-ref of="Current VI Reference"() -> (w58:refnum<vi>)
        n22 = Not(x=w65) -> (.not. x?=w62:bool)
        n23 = Equal?(x=w64, y=T3."Run Time System" ("Application:Kind")) -> (x = y?=w61:bool)
        n24 = Or(x=w62, y=w61) -> (x .or. y?=w59:bool)
        n25 = Bundle By Name(cluster=w60, "Core.Current VI Reference"=w58, "Core.Close Panel on Exit?"=w59) -> (w67:T6)
        n26 = call <vilib>:"Add State(s) to Queue__jki_lib_state_machine.vi"("State(s) in (\"\")"=w69) -> ("States Out"=w68:string)  [unwired: 14 in]
      }
      frame "Error Handler" {
        # "Unhandled Error -- Display it"
        # "Handle any errors here.\nYou can also output any states to clean-up after errors occur"
        # "Clear error"
        n27 = call <vilib>:"General Error Handler.vi"("error in (no error)"=w71) -> ()  [unwired: 10 in, 5 out]
        n28 = call <vilib>:"Add State(s) to Queue__jki_lib_state_machine.vi"("State(s) in Front (\"\")"="/* Post Error States", "State(s) in (\"\")"=w75) -> ("States Out"=w74:string)  [unwired: 13 in]
      }
      frame "Exit" {
        # "Do not put any code in this frame.\n(No errors that occur here will be handled.)"
        n29 = call <vilib>:"Add State(s) to Queue__jki_lib_state_machine.vi"("State(s) in (\"\")"=w80) -> ("States Out"=w79:string)  [unwired: 14 in]
      }
      frame "---------- DATA ----------" {
        # "Do not put any code in this frame.\n(It is a separator no-op. You can make a copy of this frame to create a new Data frame)"
        n30 = call <vilib>:"Add State(s) to Queue__jki_lib_state_machine.vi"("State(s) in (\"\")"=w84) -> ("States Out"=w83:string)  [unwired: 14 in]
      }
      frame "Data: Initialize" {
        w85 = T6 {"Core"={"Current VI Reference"=refnum, "Close Panel on Exit?"=FALSE}, "Sweep Data Cluster"={"Vfast"=[], "Vslow"=[], "Vslowest"=[], "Comments"="", "Scan names"=[]}, "Cursor Info"={"Fast Index"=[], "Slow Index"=0.0, "Slow Indices"=[], "Raw Cursor Position"={"X"=0.0, "Y"=0.0}, "Field / temp"=0}, "Scan names"=[], "Data DVR"=refnum}  # State Wire IN
        # "Data names and types of shift register data are defined by this bundle."
        # "Initialize the shift-register data, here.\n(data names are defined by what you wire into the bundle function)"
        n31 = disable-structure shown="Disabled" {
          frame Disabled {
            w90 = string[] ["DAQ_Vbg", "B", "B"]  # Scan names
            w91 = T8 {"Fast Index (Cursor X)"=[], "Slow Index (Cursor Y)"=0.0, "Slow Indices"=[], "Raw Cursor Position"={"X"=0.0, "Y"=0.0}}  # Cursor Info
            w92 = T9 {"Vfast"=[], "Vslow"=[], "Vslowest"=[], "Comments"="", "Scan names"=[]}  # Metadata Cluster
            (unwired) refnum<data-value> refnum  # Data DVR
            w93 = T10 {"Current VI Reference"=refnum, "Close Panel on Exit?"=FALSE}  # Core
            w94 = ""  # Your string data
            w95 = TRUE  # Your Boolean data
            # "do not delete - used by framework"
            n32 = Bundle("Core"=w93, "Your Boolean data"=w95, "Your string data"=w94, "Data Cell"=T4 [], "Metadata Cluster"=w92, "Cursor Info"=w91, "Scan names"=w90) -> ()  [unwired: 1 in, 1 out]
          }
          frame Enabled {
          }
        }
        n33 = call <vilib>:"Add State(s) to Queue__jki_lib_state_machine.vi"("State(s) in (\"\")"=w88) -> ("States Out"=w87:string)  [unwired: 14 in]
      }
      frame "Data: Cleanup" {
        # "Cleanup any data and references, here.\n(this is called automatically, by the Macro: Exit)"
        n34 = Unbundle By Name(w96) -> ("Core.Current VI Reference"=w99:refnum<vi>)
        n35 = Close Reference(reference=w99, error in (no error)=w98) -> (error out=w97:errorcluster)
        n36 = call <vilib>:"Add State(s) to Queue__jki_lib_state_machine.vi"("State(s) in (\"\")"=w101) -> ("States Out"=w100:string)  [unwired: 14 in]
      }
      frame "---------- UI ----------" {
        # "Do not put any code in this frame.\n(It is a separator no-op. You can make a copy of this frame to create a new UI frame)"
        n37 = call <vilib>:"Add State(s) to Queue__jki_lib_state_machine.vi"("State(s) in (\"\")"=w105) -> ("States Out"=w104:string)  [unwired: 14 in]
      }
      frame "UI: Initialize" {
        # "Initialize the User Interface, here.\n(this is called automatically, by the Macro: Init)"
        n38 = call <vilib>:"Add State(s) to Queue__jki_lib_state_machine.vi"("State(s) in (\"\")"=w109) -> ("States Out"=w108:string)  [unwired: 14 in]
      }
      frame "UI: Cursor Set" {
        # "Argument"
        # "Set and Unset Cursor Busy.\n(Usage: \"UI: Cursor Set >> Busy|Idle\")"
        n39 = case shown="\"Idle\", Default" w110 {
          tunnel: w112 -> [w117 w119]
          tunnel: [w116 w118] -> w111
          frame "Idle", Default {
            n40 = call <vilib>:"Unset Busy.vi"("error in (no error)"=w117) -> ("error out"=w116:errorcluster)  [unwired: 10 in]
          }
          frame "Busy" {
            n41 = call <vilib>:"Set Busy.vi"("error in (no error)"=w119) -> ("error out"=w118:errorcluster)  [unwired: 9 in, 1 out]
          }
        }
        n42 = call <vilib>:"Add State(s) to Queue__jki_lib_state_machine.vi"("State(s) in (\"\")"=w115) -> ("States Out"=w114:string)  [unwired: 14 in]
      }
      frame "UI: Front Panel State" {
        # "Argument"
        # "Set Front Panel Open or Closed\n(Usage: \"UI: Front Panel State >> Open|Close\")"
        n43 = Unbundle By Name(w122) -> ("Core.Current VI Reference"=w121:refnum<vi>)
        n44 = case shown="\"Open\", Default" w120 {
          tunnel: w124 -> [w130 w143]
          tunnel: [w132 w144] -> w123
          tunnel: w121 -> [w131 w141]
          frame "Open", Default {
            n45 = property class="VI"(reference=w131, error in=w130) -> (reference out=w128:refnum<vi>, error out=w129:errorcluster, "Front Panel.Open"=w127:bool)
            n46 = case shown="True" w127 {
              tunnel: [w135 w138] -> w132
              tunnel: w129 -> [w134 w138]
              tunnel: w128 -> [w133 _]
              frame False {
                n47 = invoke class="VI" method="FP.Open"(reference=w133, error in=w134, "Activate"=TRUE, "State"=T5."Standard") -> (error out=w135:errorcluster)  [unwired: 1 in, 4 out]
              }
              frame True {
              }
            }
          }
          frame "Close" {
            n48 = property class="VI"(reference=w141, error in=w143) -> (reference out=w140:refnum<vi>, error out=w142:errorcluster, "Front Panel.Open"=w139:bool)
            n49 = case shown="True" w139 {
              tunnel: [w145 w148] -> w144
              tunnel: w142 -> [w145 w147]
              tunnel: w140 -> [_ w146]
              frame False {
              }
              frame True {
                n50 = invoke class="VI" method="FP.Close"(reference=w146, error in=w147) -> (error out=w148:errorcluster)  [unwired: 1 in, 2 out]
              }
            }
          }
        }
        n51 = call <vilib>:"Add State(s) to Queue__jki_lib_state_machine.vi"("State(s) in (\"\")"=w126) -> ("States Out"=w125:string)  [unwired: 14 in]
      }
      frame "---------- Macro ----------" {
        # "Do not put any code in this frame.\n(It is a separator no-op. You can make a copy of this frame to create a new Macro frame)"
        n52 = call <vilib>:"Add State(s) to Queue__jki_lib_state_machine.vi"("State(s) in (\"\")"=w152) -> ("States Out"=w151:string)  [unwired: 14 in]
      }
      frame "Macro: Initialize" {
        # "Initialization Macro\n(This is called once, when the VI starts)"
        n53 = call <vilib>:"Add State(s) to Queue__jki_lib_state_machine.vi"("State(s) in Front (\"\")"="Data: Initialize\nInitialize Core Data\nUI: Initialize\nUI: Front Panel State >> Open\nMacro: LOAD\nMacro: Visualize", "State(s) in (\"\")"=w157) -> ("States Out"=w156:string)  [unwired: 13 in]
      }
      frame "Macro: Exit" {
        # "Exit Macro\n(This is called once, when the VI exits)"
        n54 = Unbundle By Name(w164) -> ("Core.Close Panel on Exit?"=w163:bool)
        n55 = Select(t="UI: Front Panel State >> Close", s=w163, f="") -> (s? t:f=w160:string)
        n56 = call <vilib>:"Add State(s) to Queue__jki_lib_state_machine.vi"("State(s) in (\"\")"=w160, "State(s) at Back (\"\")"="Data: Cleanup\nExit") -> ("States Out"=w158:string)  [unwired: 13 in]
        n57 = call <vilib>:"Add State(s) to Queue__jki_lib_state_machine.vi"("State(s) in Front (\"\")"=w158, "State(s) in (\"\")"=w167) -> ("States Out"=w166:string)  [unwired: 13 in]
      }
      frame "Macro: LOAD" {
        # "Exit Macro\n(This is called once, when the VI exits)"
        n58 = call <vilib>:"Add State(s) to Queue__jki_lib_state_machine.vi"("State(s) in Front (\"\")"="LOAD: Load that .dat data" ("State(s) in Front (\"\")"), "State(s) in (\"\")"=w172) -> ("States Out"=w171:string)  [unwired: 13 in]
      }
      frame "Macro: VISUALIZE" {
        # "Skip or don't skip filtering step"
        # "Exit Macro\n(This is called once, when the VI exits)"
        n59 = Select(t="VISUALIZE: Apply SG Filter", s="Filter retrieved data? 2", f="") -> (s? t:f=w177:string)
        n60 = call <vilib>:"Add State(s) to Queue__jki_lib_state_machine.vi"("State(s) in Front (\"\")"="VISUALIZE: Initialize Cursor Graph\nVISUALIZE: Initialize Color Tables" ("State(s) in Front (\"\")"), "State(s) in (\"\")"=w177, "State(s) at Back (\"\")"="//VISUALIZE: Cursor Things\nVISUALIZE: Graph Something" ("State(s) at Back (\"\")")) -> ("States Out"=w176:string)  [unwired: 12 in]
        n61 = call <vilib>:"Add State(s) to Queue__jki_lib_state_machine.vi"("State(s) in Front (\"\")"=w176, "State(s) in (\"\")"=w183) -> ("States Out"=w182:string)  [unwired: 13 in]
      }
      frame "---------- LOAD ----------" {
        # "Template Separator\n(You can make a copy of, or modify, this frame)"
        n62 = call <vilib>:"Add State(s) to Queue__jki_lib_state_machine.vi"("State(s) in (\"\")"=w187) -> ("States Out"=w186:string)  [unwired: 14 in]
      }
      frame "LOAD: Load that .dat data" {
        # "DVR"
        # "differentate and rebundle the IV data"
        # "separate meta-ish data and IV data"
        # "Read .dat file"
        n63 = call "DataVIS_Read .DAT Data.vi"("error in (no error)"=w206, "file path (use dialog)"="file path (use dialog)") -> ("error out"=w192:errorcluster, "Array"=w204:T11)  [unwired: 8 in]
        n64 = Index Array(array=w204) -> (element=w205:T12)  [unwired: 1 in]
        n65 = Unbundle By Name(w205) -> ("IV-2T"=w194:cluster{dbl[], dbl[]}[][][], "IV"=w195:cluster{dbl[], dbl[]}[][][], "Vfast"=w200:dbl[][], "Vslow"=w199:dbl[], "Vslowest"=w198:dbl[], "Comments"=w197:string, "Scan names"=w190:string[])
        "Scan names" <- w190
        n66 = Bundle("Vfast"=w200, "Vslow"=w199, "Vslowest"=w198, "Comments"=w197, "Scan names"=w190) -> (w196:T9)  [unwired: 1 in]
        n67 = call "DataVIS_Differentiate_and_Rebundle.vi"("Fit Points"="Fit Points", "error in (no error)"=w192, "IV"=w195, "IV-2T"=w194) -> ("error out"=w191:errorcluster, "Data Cell"=w189:T4)  [unwired: 6 in]
        n68 = New Data Value Reference(data value=w189, error in=w191) -> (data value reference=w188:refnum<data-value>, error out=w201:errorcluster)
        n69 = Bundle By Name(cluster=w203, "Data DVR"=w188, "Sweep Data Cluster"=w196, "Scan names"=w190) -> (w202:T6)
        n70 = call <vilib>:"Add State(s) to Queue__jki_lib_state_machine.vi"("State(s) in (\"\")"=w209) -> ("States Out"=w208:string)  [unwired: 14 in]
      }
      frame "LOAD: empty" {
        # "Your code here.\n(You can make a copy of, or modify, this frame)"
        n71 = call <vilib>:"Add State(s) to Queue__jki_lib_state_machine.vi"("State(s) in (\"\")"=w213) -> ("States Out"=w212:string)  [unwired: 14 in]
      }
      frame "---------- VISUALIZE ----------" {
        # "Template Separator\n(You can make a copy of, or modify, this frame)"
        n72 = call <vilib>:"Add State(s) to Queue__jki_lib_state_machine.vi"("State(s) in (\"\")"=w217) -> ("States Out"=w216:string)  [unwired: 14 in]
      }
      frame "VISUALIZE: Initialize Cursor Graph" {
        # "Template Separator\n(You can make a copy of, or modify, this frame)"
        n73 = Unbundle By Name(w233) -> ("Sweep Data Cluster.Vfast"=w225:dbl[][], "Sweep Data Cluster.Vslow"=w226:dbl[])  [unwired: 1 out]
        n74 = local read "Scan names"() -> (w224:string[])
        n75 = Transpose 2D Array(2D array=w225) -> (transposed array=w232:dbl[][])
        n76 = for {
          tunnel: w232 -> [w241] mode=indexing
          tunnel: [w242] -> _ mode=indexing
          tunnel: w226 -> [w238]
          shift-right: [w239] -> w229
          shift-left: dbl[] [] -> [w240]
          shift-right: [w237] -> w228
          shift-left: dbl[] [] -> [w236]
          n77 = Build Array (concatenate)(w240, w241) -> (w239:dbl[])
          n78 = Build Array (concatenate)(w236, w238) -> (w237:dbl[])
          n79 = Bundle(w241, "Vslow"=w238) -> (w242:cluster{dbl[], "Vslow":dbl[]})  [unwired: 1 in]
        }
        n80 = Index Array(array=w224, index #2=1 ("index")) -> (element #1=w222:string, element #2=w221:string)  [unwired: 1 in]
        n81 = property on="Cursor Graph" class="XYGraph (strict)"(error in=w219, "XScale.NameLbl.Text"=w222) -> (error out=w220:errorcluster)  [unwired: 1 in, 1 out]
        n82 = property on="Cursor Graph" class="XYGraph (strict)"(error in=w220, "YScale.NameLbl.Text"=w221) -> (error out=w218:errorcluster)  [unwired: 1 in, 1 out]
        n83 = Bundle(w229, w228) -> (→"Cursor Graph":cluster{dbl[], dbl[]})  [unwired: 1 in]
        n84 = call <vilib>:"Add State(s) to Queue__jki_lib_state_machine.vi"("State(s) in (\"\")"=w235) -> ("States Out"=w234:string)  [unwired: 14 in]
      }
      frame "VISUALIZE: Initialize Color Tables" {
        # "#TODO:"
        # "Set color tables"
        # "Template Separator\n(You can make a copy of, or modify, this frame)"
        n85 = Reverse 1D Array(array="color scale") -> (reversed array=w245:u32[])
        n86 = call <userlib>:"Make Color Table.vi"("Array"=w245) -> ("Color Tbl"=w243:u32[])  [unwired: 1 in, 3 out]
        n87 = property on="2term Intensity" class="IntGraph (strict)"("Color Table"=w243) -> ()  [unwired: 2 in, 2 out]
        n88 = call <vilib>:"Add State(s) to Queue__jki_lib_state_machine.vi"("State(s) in (\"\")"=w249) -> ("States Out"=w248:string)  [unwired: 14 in]
      }
      frame "VISUALIZE: Apply SG Filter" {
        # "NOT IMPLEMENTED YET\n#TODO: this"
        # "Template Separator\n(You can make a copy of, or modify, this frame)"
        n89 = call <vilib>:"Add State(s) to Queue__jki_lib_state_machine.vi"("State(s) in (\"\")"=w253) -> ("States Out"=w252:string)  [unwired: 14 in]
      }
      frame "VISUALIZE: Cursor Things" {
        # "trash if this all gets put into In-place element structure"
        # "#TODO: work out this state logic, for now just repeat\n'case 3' cursor things and graph something"
        # "Template Separator\n(You can make a copy of, or modify, this frame)"
        n90 = Unbundle By Name(w255) -> ("Sweep Data Cluster.Vfast"=w262:dbl[][], "Sweep Data Cluster.Vslow"=w261:dbl[], "Sweep Data Cluster.Vslowest"=w260:dbl[])
        n91 = disable-structure shown="Enabled" {
          disable-tunnel: w262 -> [w279 _]
          disable-tunnel: w261 -> [w278 _]
          disable-tunnel: w260 -> [w277 _]
          disable-tunnel: [w276 _] -> w259
          disable-tunnel: [w275 _] -> w258
          disable-tunnel: [w274 _] -> w257
          disable-tunnel: [w273 _] -> w256
          frame Disabled {
            n92 = Index Array(array=w277) -> (element=w267:dbl, index=w269:i32)
            n93 = Array Size(array=w277) -> (size(s)=w272:i32)
            n94 = call "DataVIS_Get_Cursor_Indices.vi"("Vslow"=w278, "Vfast"=w279) -> ("Slow Indices"=w274:dbl[], "Slow Index (Cursor Y)"=w275:dbl, "Fast Index (Cursor X) (IDK why it's an array)"=w276:dbl[], "Raw Cursor Position"=w273:T7, "Cursor Graph"=w270:refnum<vi>)  [unwired: 4 in, 1 out]
            n95 = Decrement(x=w272) -> (x-1=w271:i32)
            n96 = Unbundle By Name(w273) -> ("Y"=w266:dbl)  [unwired: 1 out]
            n97 = property on="Property Node" class="Slide (strict)"("Scale.Maximum"=w271) -> (reference=w268:refnum<vi>)  [unwired: 1 in, 2 out]
          }
          frame Enabled {
          }
        }
        n98 = disable-structure shown="Enabled" {
          frame Disabled {
            n99 = local read "side points 4Ttemp"() -> (w289:i32)
            n100 = local read "side points 2Ttemp"() -> (w290:i32)
            n101 = local read "side points 2T 2"() -> (w291:i32)
            n102 = local read "side points 4T 2"() -> (w288:i32)
            n103 = Not Equal?(x=w289, y=w288) -> (x != y?=w287:bool)
            n104 = Not Equal?(x=w291, y=w290) -> (x != y?=w286:bool)
            n105 = Or(x=w287, y=w286) -> (x .or. y?=w285:bool)
            n106 = Select(t=2, s=w285, f=3) -> (s? t:f=w280:i32)
            n107 = Select(t=4, s="stop", f=w280) -> ()  [unwired: 1 out]
          }
          frame Enabled {
          }
        }
        n108 = Bundle By Name(cluster=w255, "Cursor Info.Fast Index"=w259, "Cursor Info.Slow Index"=w258, "Cursor Info.Slow Indices"=w257, "Cursor Info.Raw Cursor Position"=w256) -> (w254:T6)
        n109 = call <vilib>:"Add State(s) to Queue__jki_lib_state_machine.vi"("State(s) in (\"\")"=w265) -> ("States Out"=w264:string)  [unwired: 14 in]
      }
      frame "VISUALIZE: Graph Something" {
        # "#TODO: if it's slow, keep the main looping INSIDE this"
        n110 = Unbundle By Name(w297) -> ("Data DVR"=w294:refnum<data-value>, "Scan names"=w301:string[], "Sweep Data Cluster.Vfast"=w293:dbl[][], "Cursor Info.Slow Index"=w292:dbl)
        n111 = in-place {
          in-place-border: w293 -> [w338]
          in-place-border: w292 -> [w337]
          in-place-border: w301 -> [w336]
          in-place-border: w297 -> [w335]
          in-place-border: [w334] -> w298
          in-place-border: [w333] -> w299
          in-place-border: w300 -> [w332]
          # "update cursor"
          # "Offset and step of fast vals"
          # "Decimate it"
          # "Select an AvsB curve"
          n112 = local read "Field/Temperature"() -> (w315:i32)
          n113 = in-place-dvr #1(w294) -> (w305:T4)  [unwired: 1 out]
          n114 = control-ref of="Cursor Graph"() -> (w316:refnum<vi>)
          n115 = control-ref of="Field/Temperature"() -> (w314:refnum<vi>)
          n116 = call "ZDataVIS_Update_Cursor_SingleArrayTest.vi"("Field/Temperature 2"=w314, "error in (no error)"=w332, "Cursor Graph"=w316, "Field / temp"=w315, "State Wire IN 2"=w335) -> ("error out"=w317:errorcluster, "Field"=→"Field":dbl, "slowest"=→"slowest":dbl, "State Wire IN 3"=w334:T6)  [unwired: 3 in]
          n117 = call "ZDataVIS_Select_Intensity.vi"("B"="Y Axis", "A"="X Axis", "error in (no error)"=w317, "Slow Index (Row)"=w337, "Slowest Index (Page)"="Field/Temperature", "Big Ol Array IN"=w305) -> ("error out"=w309:errorcluster, "Intensity Info OUT"=w303:cluster{dbl[], dbl[]}[])  [unwired: 4 in]
          n118 = Index Array(array=w336, index="Y Axis") -> (element=w324:string)
          n119 = call "ZDataVIS_ScaleSelect.vi"("Manual CTLs"="Manual CTLs", "Auto CTLs"="Auto CTLs", "error in (no error)"=w309, "X Scale Selection 2"="X Scale Selection", "Intensity Info IN"=w303) -> ("error out"=w308:errorcluster, "X Step Info"=w304:cluster{"X Low":dbl, "X High":dbl, "X Step":dbl}, "Intensity InfoOUT"=w302:cluster{dbl[], dbl[]}[])  [unwired: 4 in]
          "XY Graph" <- w302
          n120 = Index Array(array=w338, index (row)=w337) -> (element=w322:dbl[])  [unwired: 1 in]
          n121 = Unbundle By Name(w304) -> ("X Step"=w318:dbl)
          n122 = call "ZDataVIS_Offset+Multiplier.vi"("Vfast"=w322) -> ("Cluster"=w321:cluster{dbl, dbl})  [unwired: 10 in]
          n123 = call "ZDataVIS_Decimate+Fill_Intensity_Plot.vi"("Voffset -2T"="Voffset -2T", "error in (no error)"=w308, "fake point value"="Fake Point Value", "Step Info"=w304, "X and Y Arrays to decimate"=w302) -> ("error out"=w325:errorcluster, "Offset X Low"=w319:dbl, "Arr of Y arrays (intensity info)"=w320:dbl[][])  [unwired: 3 in, 1 out]
          n124 = Bundle("Offset X Low"=w319, "X Step"=w318) -> (w323:cluster{"Offset X Low":dbl, "X Step":dbl})  [unwired: 1 in]
          n125 = control-ref of="2term Intensity"() -> (w327:refnum<vi>)
          n126 = Transpose 2D Array(2D array=w320) -> (transposed array=→"2term Intensity":dbl[][])
          n127 = call "ZDataVIS_Configure_Intensity_Plot.vi"("Scan Name"=w324, "error in (no error)"=w325, "Y Offset and Multiplier"=w321, "X Offset and Multiplier"=w323, "IntensityGraph in"=w327) -> ("error out"=w333:errorcluster)  [unwired: 6 in]
          n128 = in-place-dvr #1(w305) -> ()  [unwired: 2 out]
        }
        n129 = call <vilib>:"Add State(s) to Queue__jki_lib_state_machine.vi"("State(s) in (\"\")"=w296) -> ("States Out"=w295:string)  [unwired: 14 in]
      }
    }
  }
